vi "Atomically coordinate two structures.vi"(9 "1st Pass Closeness":dbl, 10 "Second Structure":T1, 11 "First Structure":T1) -> (3 "Coordinated 2nd Structure":T1)   [LabVIEW 2010]
uses:
  <vilib>/Analysis/_algsub.llb/Real Vector Norm.vi
  <vilib>/Analysis/NI_AALPro.lvlib
panel:
  out "Array 2":dbl[][](array[numeric])
  out "Array":cluster{string, dbl[][]}[](array[cluster])
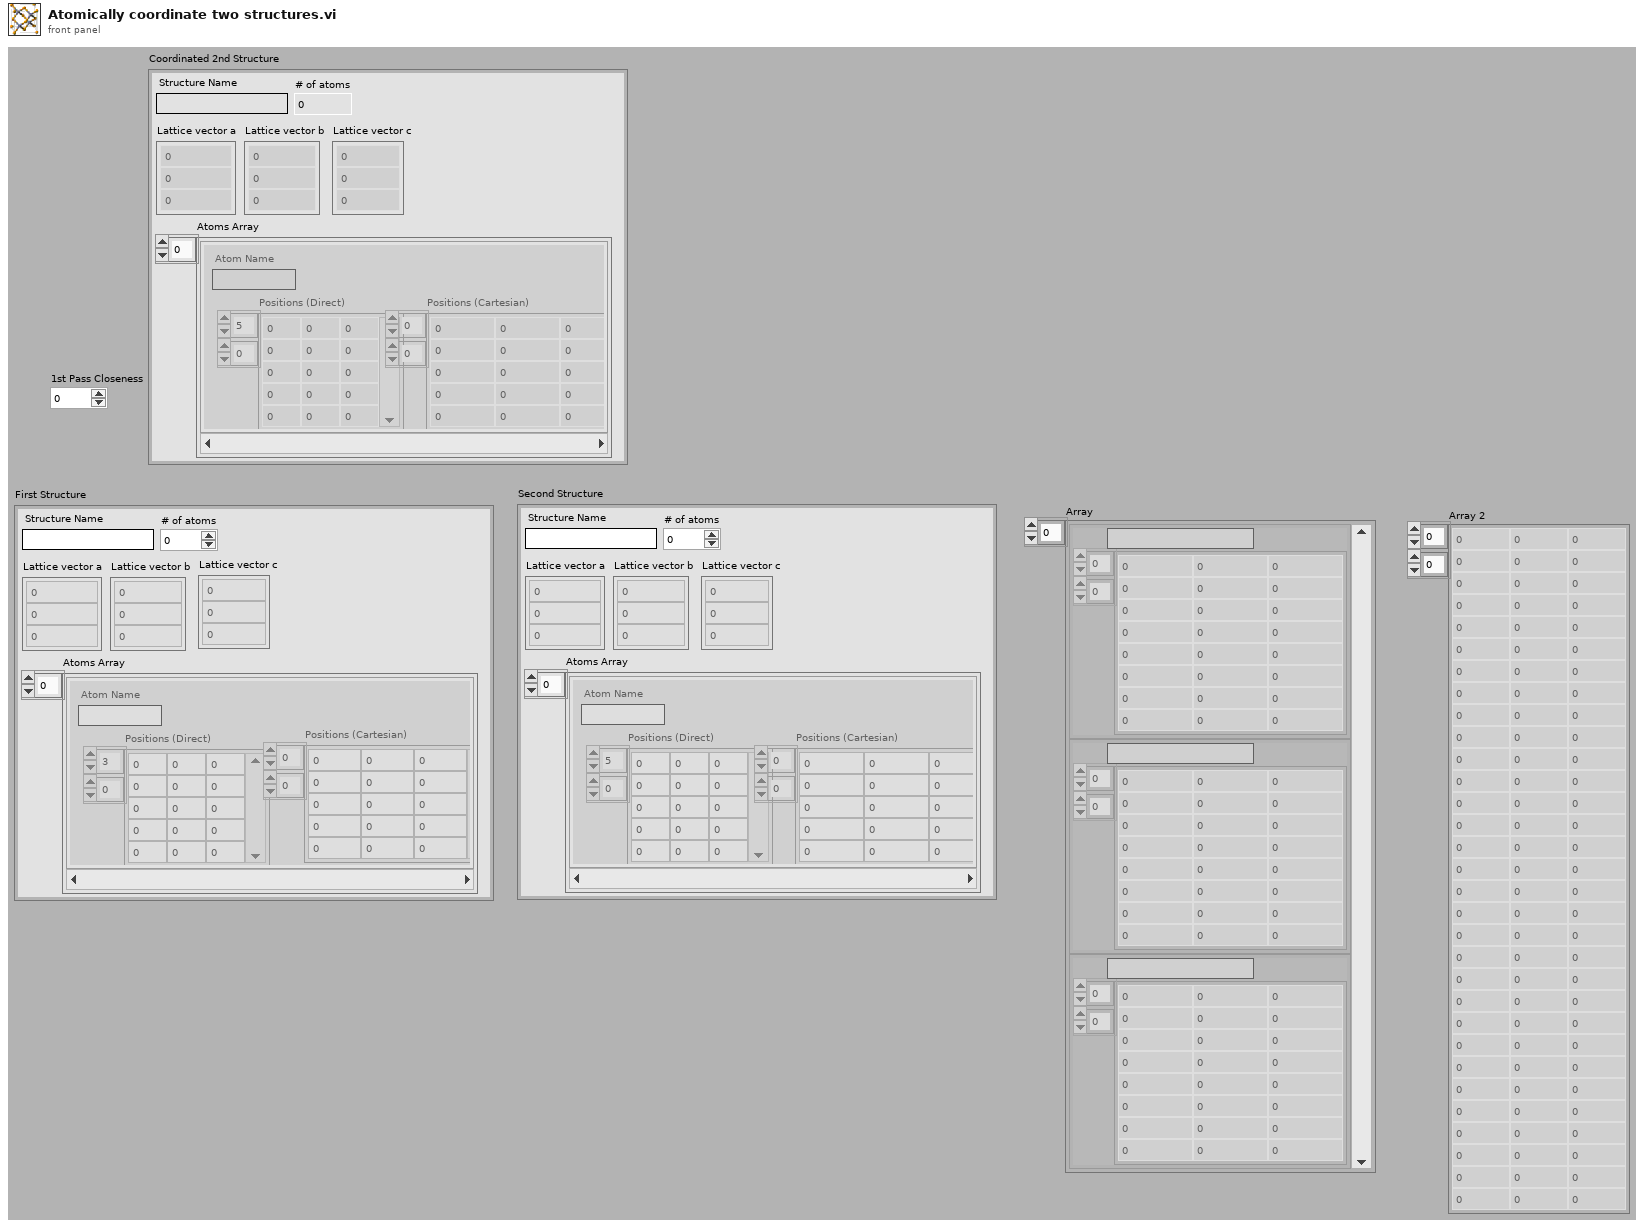
[diagram p1: front panel]
types:
  T1 = cluster{"Structure Name":string, "Lattice vector a":dbl[], "Lattice vector b":dbl[], "Lattice vector c":dbl[], "Atoms Array":cluster{"Atom Name":string, "Positions (Direct)":dbl[][], "Positions (Cartesian)":dbl[][]}[], "# of atoms":i32}
  T2 = cluster{"Atom Name":string, "Positions (Direct)":dbl[][], "Positions (Cartesian)":dbl[][]}[]
  T3 = cluster{"Atom Name":string, "Positions (Direct)":dbl[][], dbl[][]}
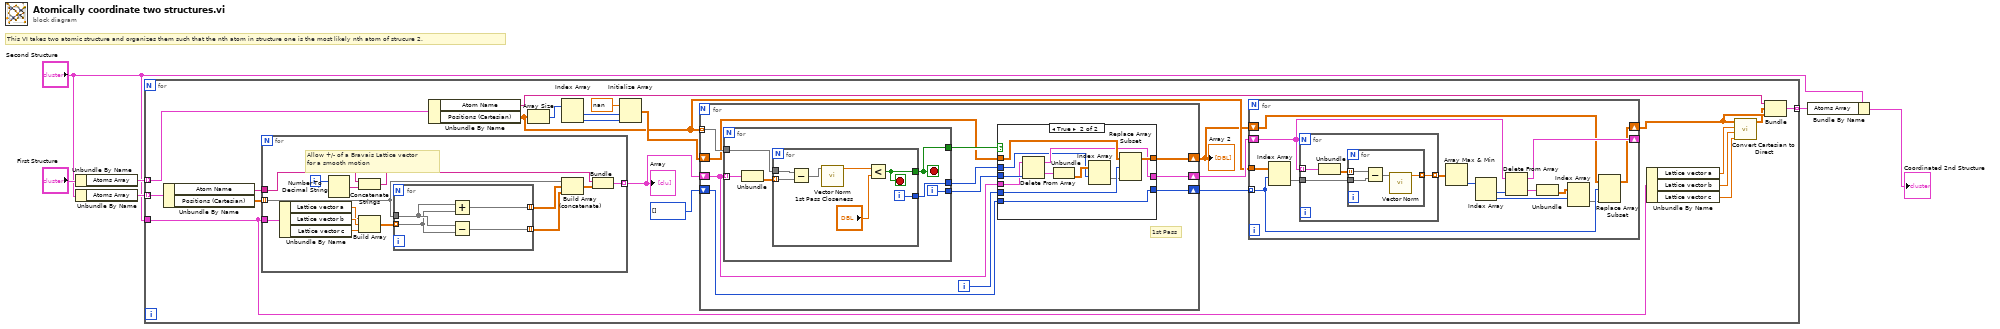
[diagram p0: block diagram]
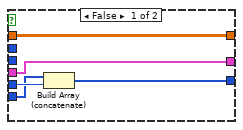
[diagram p2: hidden frame]
diagram:
  # "This VI takes two atomic structure and organizes them such that the nth atom in structure one is the most likely nth atom of strucure 2."
  n1 = Unbundle By Name("First Structure") -> ("Atoms Array"=w5:T2)
  n2 = Unbundle By Name("Second Structure") -> ("Atoms Array"=w4:T2)
  n3 = for {
    tunnel: w5 -> [w29] mode=indexing
    tunnel: w4 -> [w28] mode=indexing
    tunnel: [w25] -> w3 mode=indexing
    tunnel: "Second Structure" -> [w10]
    n4 = Unbundle By Name(w28) -> ("Atom Name"=w20:string, "Positions (Cartesian)"=w21:dbl[][])
    n5 = for {
      tunnel: w21 -> [w58] mode=indexing
      tunnel: w10 -> [w62]
      tunnel: w20 -> [w56]
      tunnel: [w52] -> w18 mode=indexing
      i -> [w55]
      # "Allow +/- of a Bravais Lattice vector\nfor a smooth motion"
      n6 = Unbundle By Name(w62) -> ("Lattice vector a"=w63:dbl[], "Lattice vector b"=w64:dbl[], "Lattice vector c"=w65:dbl[])
      n7 = Number To Decimal String(number=w55) -> (decimal integer string=w54:string)  [unwired: 1 in]
      n8 = Concatenate Strings(w56, w54) -> (w53:string)
      n9 = Build Array(w63, w64, w65) -> (w59:dbl[][])
      n10 = for {
        tunnel: w59 -> [w68] mode=indexing
        tunnel: w58 -> [w69]
        tunnel: [w67] -> w61 mode=indexing
        tunnel: [w66] -> w60 mode=indexing
        n11 = Add(x=w69, y=w68) -> (x+y=w67:dbl[])
        n12 = Subtract(x=w69, y=w68) -> (x-y=w66:dbl[])
      }
      n13 = Build Array (concatenate)(w58, w61, w60) -> (w57:dbl[][])
      n14 = Bundle(w53, w57) -> (w52:cluster{string, dbl[][]})  [unwired: 1 in]
    }
    "Array" <- w18
    n15 = Unbundle By Name(w29) -> ("Atom Name"=w26:string, "Positions (Cartesian)"=w17:dbl[][])
    n16 = Array Size(array=w17) -> (size(s)=w16:i32[])
    n17 = Index Array(array=w16) -> (element #1=w15:i32, element #2=w14:i32)  [unwired: 2 in]
    n18 = Initialize Array(nan ("element"), w15, w14) -> (w19:dbl[][])
    n19 = for {
      tunnel: w17 -> [w80] mode=indexing
      shift-right: [w75] -> w13
      shift-left: w19 -> [w77]
      shift-right: [w73] -> w22
      shift-left: w18 -> [w74]
      shift-right: [w72] -> w23
      shift-left: i32[] [] -> [w71]
      i -> [w76]
      # "1st Pass"
      n20 = for {
        tunnel: w80 -> [w102]
        tunnel: w74 -> [w99] mode=indexing
        tunnel: [w101] -> w78
        tunnel: [w100] -> w79
        tunnel: [w97] -> w70
        i -> [w101]
        stop <- w100 stop-if-true
        n21 = Unbundle(w99) -> (w98:dbl[][])  [unwired: 1 out]
        n22 = for {
          tunnel: w102 -> [w109]
          tunnel: [w104] -> w100
          tunnel: w98 -> [w105] mode=indexing
          tunnel: [w103] -> w97
          i -> [w103]
          stop <- w104 stop-if-true
          n23 = Subtract(x=w109, y=w105) -> (x-y=w108:dbl[])
          n24 = call-poly <vilib>:"Vector Norm.vi"("Input Vector"=w108) -> ("norm"=w107:dbl)  [unwired: 9 in, 1 out]
          n25 = Less?(x=w107, y="1st Pass Closeness") -> (x < y?=w104:bool)
        }
      }
      n26 = case shown="True" w79 {
        tunnel: w78 -> [_ w93]
        tunnel: w77 -> [w85 w96]
        tunnel: w76 -> [w83 w95]
        tunnel: [w85 w94] -> w75
        tunnel: w74 -> [w84 w90]
        tunnel: [w84 w92] -> w73
        tunnel: [w82 w91] -> w72
        tunnel: w71 -> [w81 w91]
        tunnel: w70 -> [_ w87]
        frame False {
          n27 = Build Array (concatenate)(w81, w83) -> (w82:i32[])
        }
        frame True {
          n28 = Delete From Array(array=w90, index=w93) -> (deleted portion=w89:cluster{string, dbl[][]}, array with subset deleted=w92:cluster{string, dbl[][]}[])  [unwired: 1 in]
          n29 = Unbundle(w89) -> (w88:dbl[][])  [unwired: 1 out]
          n30 = Index Array(array=w88, index (row)=w87) -> (element=w86:dbl[])  [unwired: 1 in]
          n31 = Replace Array Subset(array=w96, new element=w86, index (row)=w95) -> (w94:dbl[][])  [unwired: 1 in]
        }
      }
    }
    "Array 2" <- w13
    n32 = for {
      tunnel: w23 -> [w32] mode=indexing
      tunnel: w17 -> [w43]
      shift-right: [w30] -> w12
      shift-left: w13 -> [w33]
      shift-right: [w39] -> _
      shift-left: w22 -> [w40]
      n33 = Index Array(array=w43, index (row)=w32) -> (element=w42:dbl[])  [unwired: 1 in]
      n34 = for {
        tunnel: w42 -> [w45]
        tunnel: w40 -> [w47] mode=indexing
        tunnel: [w44] -> w41 mode=indexing
        n35 = Unbundle(w47) -> (w46:dbl[][])  [unwired: 1 out]
        n36 = for {
          tunnel: w46 -> [w50] mode=indexing
          tunnel: w45 -> [w49]
          tunnel: [w48] -> w44 mode=indexing
          n37 = Subtract(x=w50, y=w49) -> (x-y=w51:dbl[])
          n38 = call-poly <vilib>:"Vector Norm.vi"("Input Vector"=w51) -> ("norm"=w48:dbl)  [unwired: 9 in, 1 out]
        }
      }
      n39 = Array Max & Min(array=w41) -> (min index (indices)=w36:i32[])  [unwired: 3 out]
      n40 = Index Array(array=w36) -> (element #1=w35:i32, element #2=w34:i32)  [unwired: 2 in]
      n41 = Delete From Array(array=w40, index=w35) -> (deleted portion=w38:cluster{string, dbl[][]}, array with subset deleted=w39:cluster{string, dbl[][]}[])  [unwired: 1 in]
      n42 = Unbundle(w38) -> (w37:dbl[][])  [unwired: 1 out]
      n43 = Index Array(array=w37, index (row)=w34) -> (element=w31:dbl[])  [unwired: 1 in]
      n44 = Replace Array Subset(array=w33, new element=w31, index (row)=w32) -> (w30:dbl[][])  [unwired: 1 in]
    }
    n45 = Unbundle By Name(w10) -> ("Lattice vector a"=w9:dbl[], "Lattice vector b"=w8:dbl[], "Lattice vector c"=w7:dbl[])
    n46 = call "Convert Cartesian to Direct.vi"("Lattice vector c"=w7, "Lattice vector b"=w8, "Lattice vector a"=w9, "Positions (Cartesian)"=w12) -> ("Positions (Direct)"=w11:dbl[][])  [unwired: 7 in]
    n47 = Bundle("Atom Name"=w26, "Positions (Direct)"=w11, w12) -> (w25:T3)  [unwired: 1 in]
  }
  n48 = Bundle By Name(cluster="Second Structure", "Atoms Array"=w3) -> (→"Coordinated 2nd Structure":T1)
